vi "Get Attributes Tree Data.vi"(7 "Tree ID":string, 8 "Error In":errorcluster, 10 "Attributes Names":string[](array[string]), 11 "Tree Manager":refnum<data-value>) -> (0 "Error Out":errorcluster, 1 "Attributes Values":refnum<class "Tree Data.lvclass">[](array[class]), 2 "Found?":bool[](array[boolean]), 3 "Tree Manager":refnum<data-value>)   [LabVIEW 2017, in "Tree API.lvlib" / "Tree.lvclass"]
doc: "Get Tree Data attributes of the Tree."
uses:
  Tree.lvclass
  Tree Data/Tree Data.lvclass
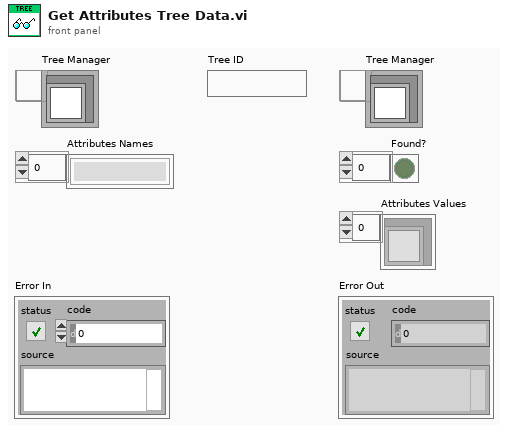
[diagram p1: front panel]
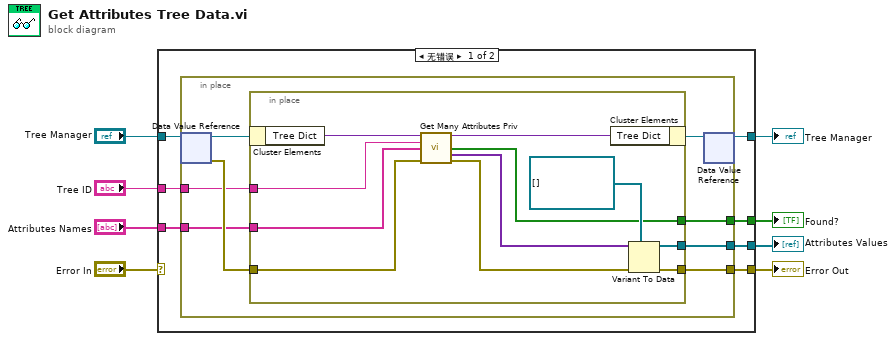
[diagram p0: block diagram]
diagram:
  n1 = case shown="无错误" "Error In" {
    selector: "Error In" -> [_ w35]
    tunnel: "Tree Manager" -> [w15 w36]
    tunnel: [w14 w36] -> w7
    tunnel: [w13 w35] -> w5
    tunnel: "Tree ID" -> [w12 _]
    tunnel: "Attributes Names" -> [w11 _]
    tunnel: [w10 _] -> w2
    tunnel: [w9 _] -> w1
    frame No Error {
      n2 = in-place {
        in-place-border: [w22] -> w13
        in-place-border: w12 -> [w19]
        in-place-border: w11 -> [w18]
        in-place-border: [w17] -> w10
        in-place-border: [w16] -> w9
        n3 = in-place-dvr #1(w15) -> (w23:refnum<class "Tree.lvclass">, w20:errorcluster)
        n4 = in-place {
          in-place-border: [w34] -> w22
          in-place-border: w20 -> [w27]
          in-place-border: w19 -> [w29]
          in-place-border: w18 -> [w28]
          in-place-border: [w25] -> w17
          in-place-border: [w32] -> w16
          n5 = in-place-cluster #2(w23) -> ("Tree Dict"=w31:variant)
          n6 = call "Get Many Attributes Priv.vi"("Tree Dictionary In"=w31, "Unique ID"=w29, "Attribute Names"=w28, "error in"=w27) -> ("Tree Dictionary Out"=w30:variant, "Found?"=w25:bool[], "Attribute Values"=w24:variant[], "error out"=w26:errorcluster)  [unwired: 6 in, 2 out]
          n7 = in-place-cluster #2("Tree Dict"=w30) -> (w21:refnum<class "Tree.lvclass">)
          n8 = Variant To Data(error in=w26, type=refnum<class "Tree Data.lvclass">[] [] ("Array"), Variant=w24) -> (data=w32:refnum<class "Tree Data.lvclass">[], error out=w34:errorcluster)
        }
        n9 = in-place-dvr #1(w21) -> (w14:refnum<data-value>)  [unwired: 1 out]
      }
    }
    frame Error {
    }
  }
  "Tree Manager" <- w7
  "Error Out" <- w5
  "Found?" <- w2
  "Attributes Values" <- w1
